vi "Actor Core.vi"(8 "error in":errorcluster, 11 "Application Manager in":refnum<class "Application Manager.lvclass">) -> (0 "error out":errorcluster, 3 "Actor out":refnum<class "Actor.lvclass">)   [LabVIEW 2020, in "Application Manager.lvlib" / "Application Manager.lvclass"]
doc: "<p>(<strong>Filename</strong>: <span class=\"dnl\">Actor Framework.lvlib:Actor.lvclass:Actor Core.vi</span>)</p>\n<p>Receives messages to the actor, reacts to them, and initiates any error handling that may shut the actor down.</p>\n<p>Descendant classes may override this VI to append parallel tasks for the actor to complete while it handles messages. Overrides use the <a href=\"nihelplauncher://docs/csh?context=lvcore_glang_udclass\">Call Parent Class Method</a> node.</p>"
uses:
  Application Manager.lvclass
  C:/Program Files/National Instruments/LabVIEW 2025/vi.lib/ActorFramework/Actor/Actor.lvclass
  <vilib>/ActorFramework/Actor/Actor.lvclass
  RFSA DAQ/RFSA DAQ/RFSA DAQ.lvclass
  C:/Users/natan/Documents/G2CPU-RTSA-Demo/Application/DAQ Interface/DAQ Interface/DAQ Interface.lvclass
  TDMS DAQ/TDMS DAQ/TDMS DAQ.lvclass
  Signal Analysis/Signal Analysis/Signal Analysis.lvclass
  UI/UI Root/UI Root/UI Root.lvclass
  C:/Program Files/National Instruments/LabVIEW 2025/vi.lib/MGI/Panel Manager/Panel Actor/Panel Actor/Panel Actor.lvclass
  Signal Analysis/Signal Analysis/Process Data.ctl
  <vilib>/Natan Biesmans/G2CPU GPU and CPU HPC Toolkit/G2CPU Libraries/Arrays/1DArray/s16/1D Array s16.lvclass
  Signal Analysis/Signal Analysis/FFT Size.ctl
  Signal Analysis/Signal Analysis Messages/Set FFT Size Msg/Set FFT Size Msg.lvclass/Set FFT Size Msg.ctl
  <vilib>/ActorFramework/Message Enqueuer/Message Enqueuer.lvclass/Message Enqueuer.ctl
  Application Manager.lvclass/Application Manager.ctl
  <vilib>/MGI/Panel Manager/Panel/Panel/Window/Window_Top Level.vi
  <vilib>/ActorFramework/Message Enqueuer/Enqueue.vi
  <vilib>/MGI/Panel Manager/Panel/Window Position/Window Position Selector.vi
  <vilib>/MGI/Panel Manager/Panel/Window Position/Maximize/Maximize.vi
  Signal Analysis/Signal Analysis Messages/Set FFT Size Msg/Set FFT Size Msg.lvclass
  C:/Program Files/National Instruments/LabVIEW 2025/vi.lib/ActorFramework/Message/Message.lvclass
  <vilib>/MGI/Panel Manager/Panel/Window Position/Maximize/Maximize.lvclass
  C:/Program Files/National Instruments/LabVIEW 2025/vi.lib/MGI/Panel Manager/Panel/Window Position/Window Position.lvclass
  <vilib>/MGI/Panel Manager/Panel/Panel/Window/Window.lvclass
  C:/Program Files/National Instruments/LabVIEW 2025/vi.lib/MGI/Panel Manager/Panel/Panel/Panel.lvclass
  <vilib>/ActorFramework/Message Priority Queue/Priority Enqueue.vi
  <vilib>/MGI/Panel Manager/Panel/Window Position/Reference Position/Ref Display/Ref Display.vi
  <vilib>/MGI/Panel Manager/Panel/Panel/Window/Window_protected.vi
  <vilib>/MGI/Panel Manager/Panel Actor/Panel Actor/Launch as Nested Actor.vi
  Primitive/Primitive/Primitive.lvclass
  C:/Users/natan/Documents/G2CPU-RTSA-Demo/Application/Primitive/Primitive/Primitive.lvclass
  C:/Program Files/National Instruments/LabVIEW 2025/vi.lib/MGI/Monitored Actor/Monitored Actor/Monitored Actor/Monitored Actor.lvclass
  C:/Users/natan/Documents/G2CPU-RTSA-Demo/Application/Application Manager/Application Manager/Application Manager.lvclass
  C:/Program Files/National Instruments/LabVIEW 2025/vi.lib/MGI/Panel Manager/Panel/Panel/Window/Window.lvclass
  C:/Users/natan/Documents/G2CPU-RTSA-Demo/Application/UI/UI Root/UI Root/UI Root.lvclass
  <vilib>/MGI/Panel Manager/Panel Actor/Panel Actor/Panel Actor.lvclass
  <vilib>/MGI/Panel Manager/Panel/Panel.lvlib
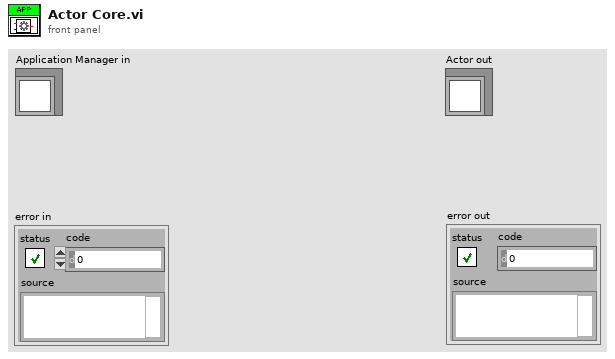
[diagram p1: front panel]
types:
  T1 = typedef "Signal Analysis.lvlib/Signal Analysis.lvclass/FFT Size.ctl" = cluster{"FFT Size":i32}
  T2 = typedef "Signal Analysis.lvlib/Signal Analysis.lvclass/Process Data.ctl" = cluster{"Gain":dbl, "dt":dbl, "Serial IQ Data":refnum<class "1D Array s16.lvclass">, "f0":dbl}
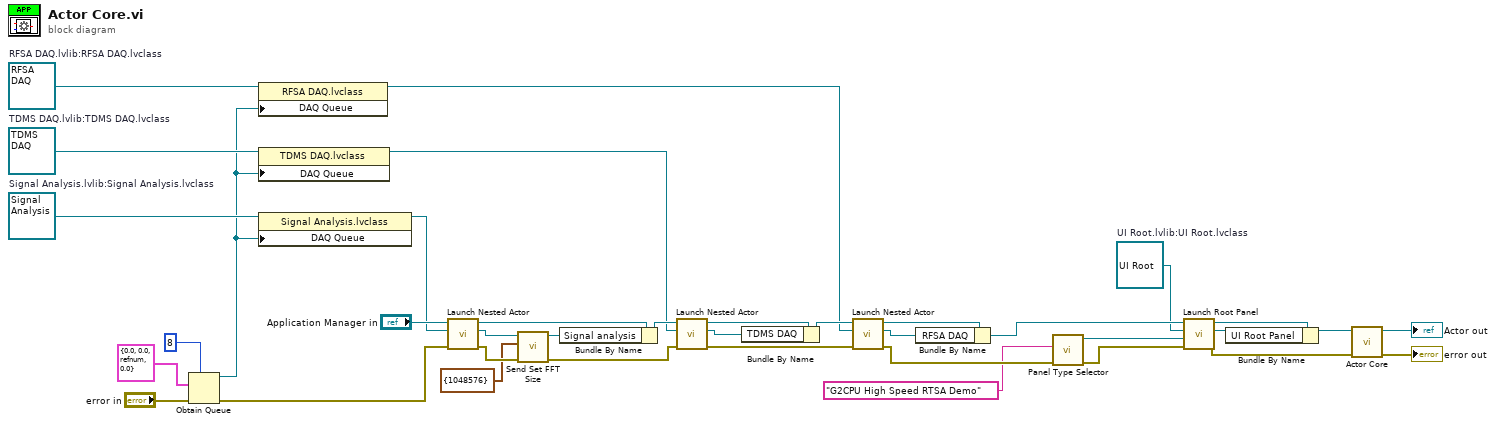
[diagram p0: block diagram]
diagram:
  w11 = refnum<class "UI Root.lvclass"> refnum  # UI Root.lvlib:UI Root.lvclass
  w32 = refnum<class "Signal Analysis.lvclass"> refnum  # Signal Analysis.lvlib:Signal Analysis.lvclass
  w31 = refnum<class "TDMS DAQ.lvclass"> refnum  # TDMS DAQ.lvlib:TDMS DAQ.lvclass
  w30 = refnum<class "RFSA DAQ.lvclass"> refnum  # RFSA DAQ.lvlib:RFSA DAQ.lvclass
  n1 = Obtain Queue(max queue size (-1, unlimited)=8, element data type=T2 {"Gain"=0.0, "dt"=0.0, "Serial IQ Data"=refnum, "f0"=0.0} ("Filled Buffers"), error in (no error)="error in") -> (queue out=w18:refnum<queue>, error out=w23:errorcluster)  [unwired: 2 in, 1 out]
  n2 = property class="RFSA DAQ.lvclass"(reference=w30, "DAQ Queue"=w18) -> (reference out=w21:refnum<class "RFSA DAQ.lvclass">)  [unwired: 1 in, 1 out]
  n3 = property class="TDMS DAQ.lvclass"(reference=w31, "DAQ Queue"=w18) -> (reference out=w20:refnum<class "TDMS DAQ.lvclass">)  [unwired: 1 in, 1 out]
  n4 = property class="Signal Analysis.lvclass"(reference=w32, "DAQ Queue"=w18) -> (reference out=w19:refnum<class "Signal Analysis.lvclass">)  [unwired: 1 in, 1 out]
  n5 = call <vilib>:"Launch Nested Actor.vi"("error in (no error)"=w23, "Nested Actor"=w19, "Caller Actor in"="Application Manager in") -> ("error out"=w5:errorcluster, "Nested Actor's Enqueuer"=w3:refnum<class "Message Enqueuer.lvclass">, "Caller Actor out"=w36:refnum<class "Application Manager.lvclass">)  [unwired: 6 in]
  n6 = call "Send Set FFT Size.vi"("error in (no error)"=w5, "FFT Size"=T1 {"FFT Size"=1048576}, "Message Enqueuer"=w3) -> ("error out"=w2:errorcluster, "Message Enqueuer out"=w1:refnum<class "Message Enqueuer.lvclass">)  [unwired: 7 in]
  n7 = Bundle By Name(cluster=w36, "Signal analysis"=w1) -> (w29:refnum<class "Application Manager.lvclass">)
  n8 = call <vilib>:"Launch Nested Actor.vi"("error in (no error)"=w2, "Nested Actor"=w20, "Caller Actor in"=w29) -> ("error out"=w34:errorcluster, "Nested Actor's Enqueuer"=w26:refnum<class "Message Enqueuer.lvclass">, "Caller Actor out"=w35:refnum<class "Application Manager.lvclass">)  [unwired: 6 in]
  n9 = Bundle By Name(cluster=w35, "TDMS DAQ"=w26) -> (w28:refnum<class "Application Manager.lvclass">)
  n10 = call <vilib>:"Launch Nested Actor.vi"("error in (no error)"=w34, "Nested Actor"=w21, "Caller Actor in"=w28) -> ("error out"=w9:errorcluster, "Nested Actor's Enqueuer"=w27:refnum<class "Message Enqueuer.lvclass">, "Caller Actor out"=w33:refnum<class "Application Manager.lvclass">)  [unwired: 6 in]
  n11 = Bundle By Name(cluster=w33, "RFSA DAQ"=w27) -> (w14:refnum<class "Application Manager.lvclass">)
  n12 = call-poly <vilib>:"Panel Type Selector.vi"("error in (no error)"=w9, "Default Title"="G2CPU High Speed RTSA Demo") -> ("error out"=w8:errorcluster, "Window out"=w10:refnum<class "Window.lvclass">)  [unwired: 8 in]
  n13 = call-poly <vilib>:"Launch Root Panel.vi"("Error In"=w8, "Panel"=w10, "Panel Actor in"=w11, "Caller Actor in"=w14) -> ("Error Out"=w17:errorcluster, "Actor's Enqueuer"=w16:refnum<class "Message Enqueuer.lvclass">, "Caller Actor out"=w12:refnum<class "Application Manager.lvclass">)  [unwired: 5 in]
  n14 = Bundle By Name(cluster=w12, "UI Root Panel"=w16) -> (w13:refnum<class "Application Manager.lvclass">)
  n15 = call-parent "Actor Core.vi"("error in"=w17, "Actor in"=w13) -> ("error out"=→"error out":errorcluster, "Actor out"=→"Actor out":refnum<class "Actor.lvclass">)  [unwired: 8 in]
